vi "Start Car Wash.vi"(8 "error in (no error)":errorcluster, 10 "Options":string[](array[string]), 11 "Car Wash Model in":refnum<class "Car Wash Model.lvclass">) -> (0 "error out":errorcluster, 3 "Car Wash Model out":refnum<class "Car Wash Model.lvclass">)   [LabVIEW 2019, in "Car Wash Model.lvclass"]
uses:
  <vilib>/gpm_packages/@cs/Car-wash/Source/Car Wash Model/Car Wash Model/Car Wash Model.lvclass
  C:/Program Files/National Instruments/LabVIEW 2019/vi.lib/gpm_packages/@cs/mva-core/Source/IModel/IModel/IModel.lvclass
  <vilib>/gpm_packages/@cs/Car-wash/Source/Car Wash Model/Car Wash Model/Car Wash Model.lvclass/Car Wash Model.ctl
  <vilib>/gpm_packages/@cs/Car-wash/Source/iProcess Model/iProcess Model Messages/Create Process Msg/Create Process Msg.lvclass/Create Process Msg.ctl
  <vilib>/ActorFramework/Message Enqueuer/Message Enqueuer.lvclass/Message Enqueuer.ctl
  <vilib>/gpm_packages/@cs/mva-core/Source/IMediator/ISubscriptionPolicy/ISubscriptionPolicy.lvclass/ISubscriptionPolicy.ctl
  <vilib>/gpm_packages/@cs/mva-core/Source/IObserver/IObserver/IObserver.lvclass/IObserver.ctl
  <vilib>/gpm_packages/@cs/mva-core/Source/IModel/IModel/IModel.lvclass/IModel.ctl
  <vilib>/gpm_packages/@cs/mva-core/Source/IMediator/PublishRequest/PublishRequest.lvclass/PublishRequest.ctl
  <vilib>/gpm_packages/@cs/mva-core/Source/IMediator/IMediator Messages/Publish Msg/Publish Msg.lvclass/Publish Msg.ctl
  <vilib>/gpm_packages/@cs/actor-framework-messages/Source/RoundTripMessage/RoundTripMessage.lvclass/RoundTripMessage.ctl
  <vilib>/ActorFramework/Message Enqueuer/Enqueue.vi
  <vilib>/gpm_packages/@cs/mva-core/Source/IMediator/IMediator Messages/Publish Msg/Send Pre-Addressed Publish.vi
  <vilib>/gpm_packages/@cs/mva-core/Source/IObserver/IObserver/Read Unique ID.vi
  <vilib>/gpm_packages/@cs/mva-core/Source/IMediator/PublishRequest/Pack Publish Request.vi
  <vilib>/gpm_packages/@cs/actor-framework-messages/Source/RoundTripMessage/Return Round-Trip Message.vi
  <vilib>/gpm_packages/@cs/Car-wash/Source/iProcess Model/iProcess Model/iProcess Model.lvclass
  <vilib>/gpm_packages/@cs/Car-wash/Source/iProcess Model/iProcess Model Messages/Create Process Msg/Create Process Msg.lvclass
  C:/Program Files/National Instruments/LabVIEW 2019/vi.lib/ActorFramework/Message/Message.lvclass
  <vilib>/gpm_packages/@cs/Car-wash/Source/iProcess Model/iProcess Model Messages/Start Process Msg/Start Process Msg.lvclass
  <vilib>/gpm_packages/@cs/mva-core/Source/IModel/IModel/IModel.lvclass
  C:/Program Files/National Instruments/LabVIEW 2019/vi.lib/gpm_packages/@cs/mva-core/Source/IObserver/IObserver/IObserver.lvclass
  <vilib>/gpm_packages/@cs/mva-core/Source/IMediator/IMediator Messages/Publish Msg/Publish Msg.lvclass
  C:/Program Files/National Instruments/LabVIEW 2019/vi.lib/gpm_packages/@cs/actor-framework-messages/Source/RoundTripMessage/RoundTripMessage.lvclass
  <vilib>/gpm_packages/@cs/actor-framework-messages/Source/RoundTripMessage/RoundTripMessage.lvclass
  <vilib>/ActorFramework/Message Priority Queue/Priority Enqueue.vi
  <vilib>/Utility/error.llb/Error Cluster From Error Code.vi
  <vilib>/gpm_packages/@cs/mva-core/Source/IMediator/PublishRequest/PublishRequest.lvclass
  <vilib>/gpm_packages/@cs/mva-core/Source/IMediator/ISubscriptionPolicy/ISubscriptionPolicy.lvclass
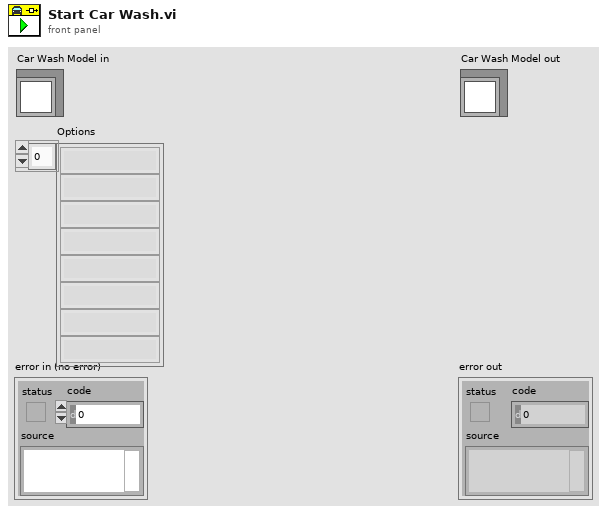
[diagram p1: front panel]
types:
  T1 = typedef "IMediator.lvlib/ISubscriptionPolicy.lvclass/ISubscriptionPolicy Reference.ctl" = refnum<data-value>
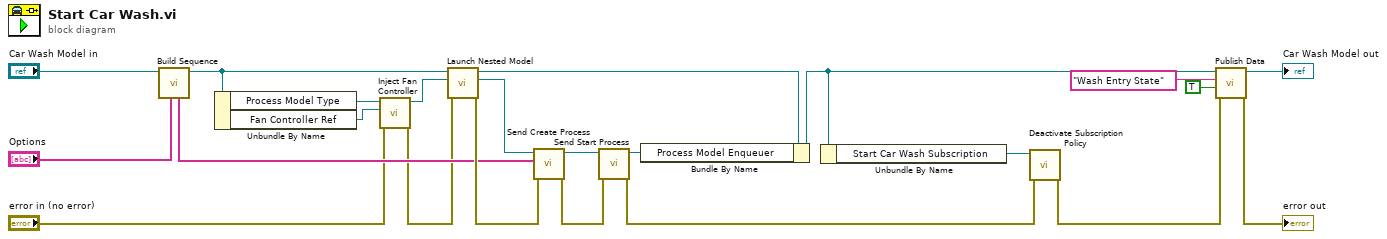
[diagram p0: block diagram]
diagram:
  n1 = call <vilib>:"Build Sequence.vi"("Options"="Options", "Car Wash Model in"="Car Wash Model in") -> ("Car Wash Model out"=w18:refnum<class "Car Wash Model.lvclass">, "Sequence"=w16:string[])  [unwired: 8 in]
  n2 = Unbundle By Name(w18) -> ("Process Model Type"=w5:refnum<class "iProcess Model.lvclass">, "Fan Controller Ref"=w3:refnum<data-value>)
  n3 = call-dynamic "Inject Fan Controller.vi"("error in (no error)"="error in (no error)", "Fan Controller Ref"=w3, "iProcess Model in"=w5) -> ("error out"=w1:errorcluster, "iProcess Model out"=w4:refnum<class "iProcess Model.lvclass">)  [unwired: 7 in]
  n4 = call-dynamic "Launch Nested Model.vi"("error in (no error)"=w1, "Model to Launch"=w4, "IModel in"=w18) -> ("error out"=w22:errorcluster, "Nested Model Enqueuer"=w23:refnum<class "Message Enqueuer.lvclass">, "IModel out"=w21:refnum<class "Car Wash Model.lvclass">)  [unwired: 6 in]
  n5 = call <vilib>:"Send Create Process.vi"("error in (no error)"=w22, "Sequence"=w16, "Message Enqueuer"=w23) -> ("error out"=w13:errorcluster, "Message Enqueuer out"=w15:refnum<class "Message Enqueuer.lvclass">)  [unwired: 7 in]
  n6 = call <vilib>:"Send Start Process.vi"("error in (no error)"=w13, "Message Enqueuer"=w15) -> ("error out"=w12:errorcluster, "Message Enqueuer out"=w14:refnum<class "Message Enqueuer.lvclass">)  [unwired: 8 in]
  n7 = Bundle By Name(cluster=w21, "Process Model Enqueuer"=w14) -> (w11:refnum<class "Car Wash Model.lvclass">)
  n8 = Unbundle By Name(w11) -> ("Start Car Wash Subscription"=w20:T1)
  n9 = call <vilib>:"Deactivate Subscription Policy.vi"("error in (no error)"=w12, "Subscription Policy"=w20) -> ("error out"=w9:errorcluster)  [unwired: 9 in]
  n10 = call <vilib>:"Publish Data.vi"("error in (no error)"=w9, "Data to Publish"=TRUE, "Datum Name"="Wash Entry State" ("Datum Name (\"\"=Use Control Label)"), "IModel in"=w11) -> ("error out"=→"error out":errorcluster, "IModel out"=→"Car Wash Model out":refnum<class "Car Wash Model.lvclass">)  [unwired: 6 in]
